vi "Delete Child.vi"(8 "error in (no error)":errorcluster, 9 "Position":i32[](array[numeric]), 10 "Tree In":refnum<class "Tree.lvclass">, 11 "Tree Data in":refnum<class "Tree Data.lvclass">) -> (0 "error out":errorcluster, 1 "Delete Child Out":refnum<class "Tree Data.lvclass">, 2 "Tree Out":refnum<class "Tree.lvclass">, 3 "Tree Data out":refnum<class "Tree Data.lvclass">)   [LabVIEW 2022 SP3, in "Tree Data.lvclass"]
uses:
  Tree Data.lvclass
  Tree/Tree.lvclass
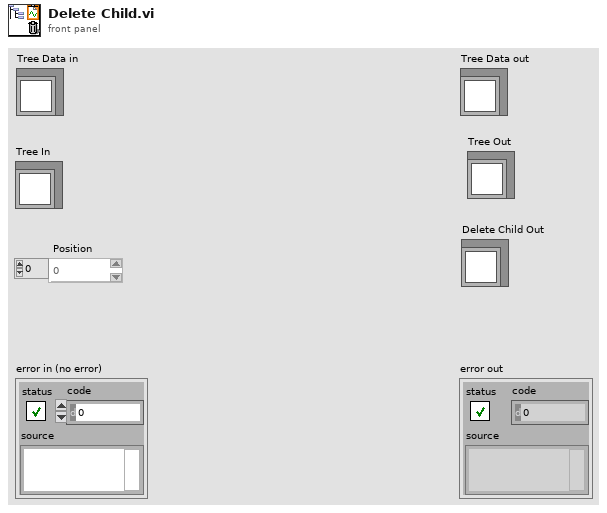
[diagram p1: front panel]
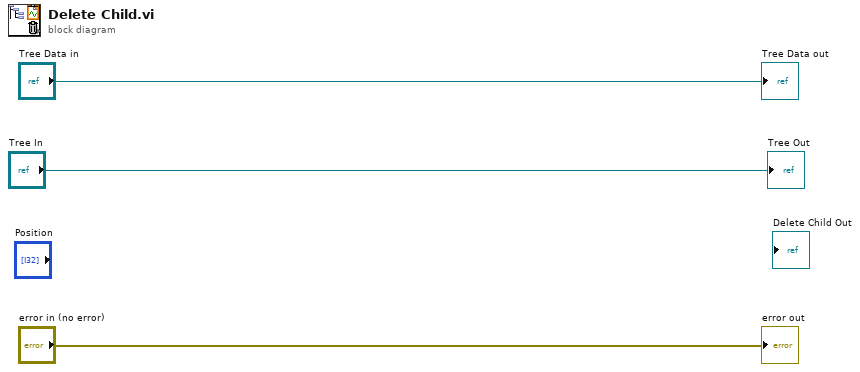
[diagram p0: block diagram]
diagram:
  "error out" <- "error in (no error)"
  "Tree Data out" <- "Tree Data in"
  "Tree Out" <- "Tree In"
